vi "Add_Endpoint.vi"(8 "error in (no error)":errorcluster, 10 "Endpoint URL":string, 11 "Request in":refnum<class "Request.lvclass">) -> (0 "error out":errorcluster, 3 "Request out":refnum<class "Request.lvclass">)   [LabVIEW 2016, in "Request.lvclass"]
uses:
  Request.lvclass
  <vilib>/Utility/error.llb/whitespace.ctl
  Request.lvclass/Request.ctl
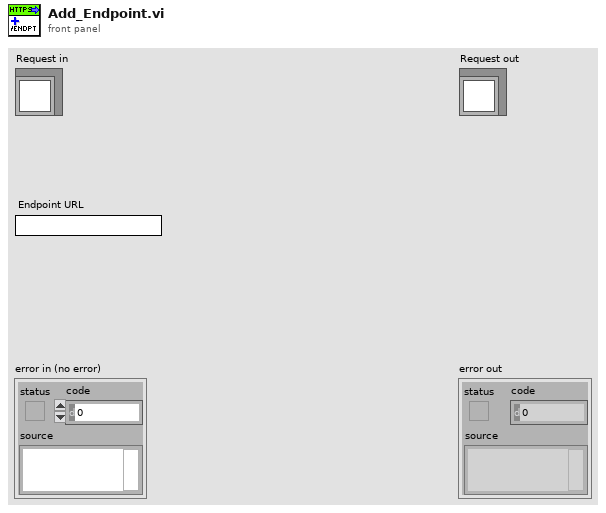
[diagram p1: front panel]
types:
  T1 = typedef "whitespace.ctl" = u16
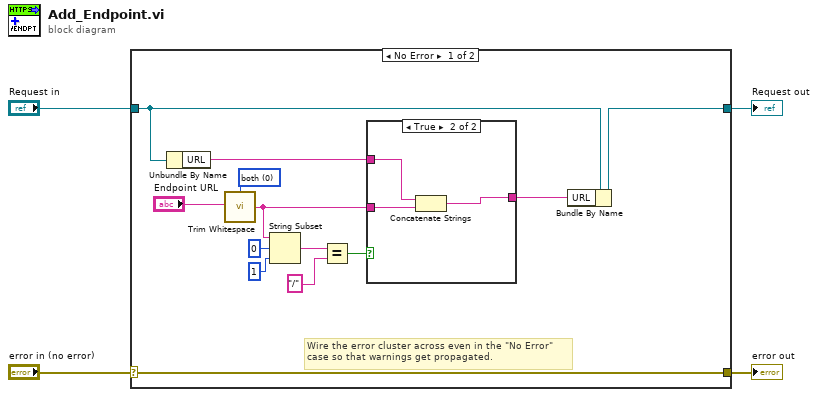
[diagram p0: block diagram]
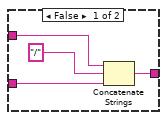
[diagram p2: hidden frame]
diagram:
  n1 = case shown="No Error" "error in (no error)" {
    selector: "error in (no error)" -> [w17 w26]
    tunnel: [w17 w26] -> w3
    tunnel: [w5 w25] -> w1
    tunnel: "Request in" -> [w6 w25]
    frame No Error {
      w15 = T1 0 items=["both", "start of string", "end of string"] ("location (both)")
      # "Wire the error cluster across even in the \"No Error\"\ncase so that warnings get propagated."
      n2 = Unbundle By Name(w6) -> ("URL"=w9:string)
      n3 = call <vilib>:"Trim Whitespace.vi"("string"="Endpoint URL", "location (both)"=w15) -> ("trimmed string"=w8:string)
      n4 = String Subset(string=w8, offset (0)=0, length (rest)=1 ("length (rest)")) -> (substring=w11:string)
      n5 = Equal?(x=w11, y="/") -> (x = y?=w10:bool)
      n6 = case shown="True" w10 {
        tunnel: [w20 w22] -> w7
        tunnel: w9 -> [w18 w24]
        tunnel: w8 -> [w19 w23]
        frame False {
          n7 = Concatenate Strings(w18, "/" ("string"), w19) -> (w20:string)
        }
        frame True {
          n8 = Concatenate Strings(w24, w23) -> (w22:string)
        }
      }
      n9 = Bundle By Name(cluster=w6, "URL"=w7) -> (w5:refnum<class "Request.lvclass">)
    }
    frame Error {
    }
  }
  "error out" <- w3
  "Request out" <- w1
